vi "3. State Machine Based Traffic Light Simulator.vi"() -> ()   [LabVIEW 2018]
uses:
  Typedefs/States for State Machine based Example.ctl
panel:
  in  "stop":bool
  out "Yellow":bool
  out "Green":bool
  out "Red":bool
  out "Traffic Lights Picture":picture
  # "Traffic Light Graphic Vector by Vecteezy\n(https://www.vecteezy.com/free-vector/graphic)"
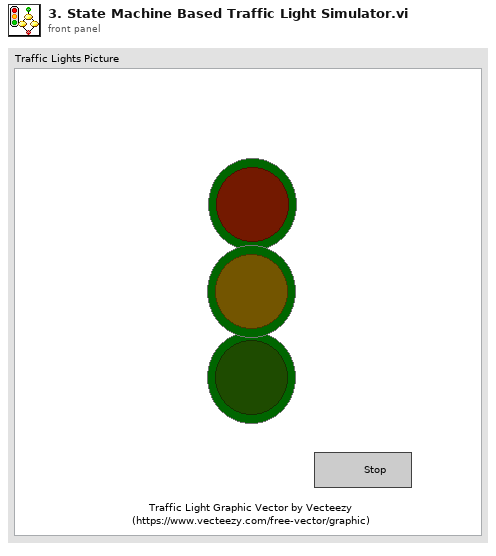
[diagram p1: front panel]
types:
  T1 = cluster{"Wait Before Red":u32, "Wait Before Yellow":u32, "Wait Before Green":u32}
  T2 = typedef "States for State Machine based Example.ctl" = enum16{"Initialize", "Red", "Yellow", "Green", "Wait Before Red", "Wait Before Yellow", "Wait Before Green", "Stop"}
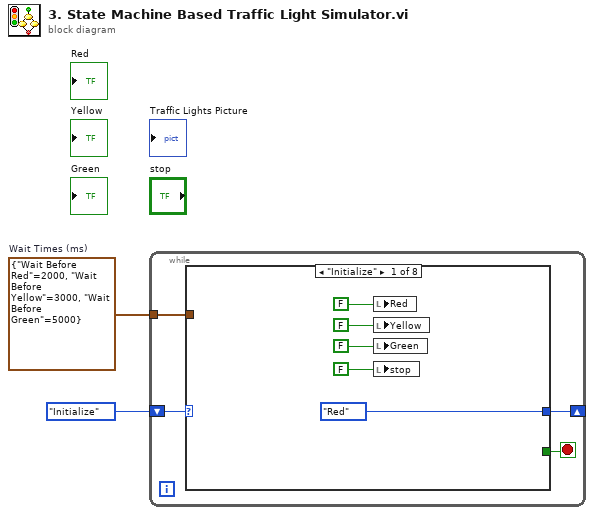
[diagram p0: block diagram]
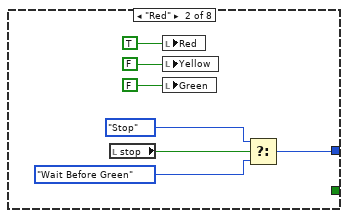
[diagram p2: hidden frame]
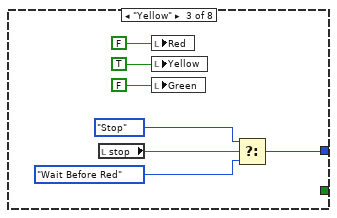
[diagram p3: hidden frame]
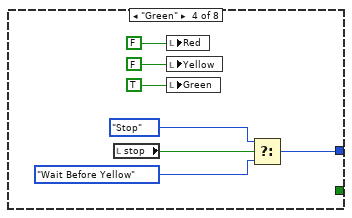
[diagram p4: hidden frame]
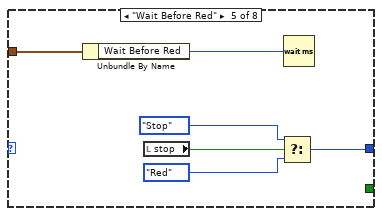
[diagram p5: hidden frame]
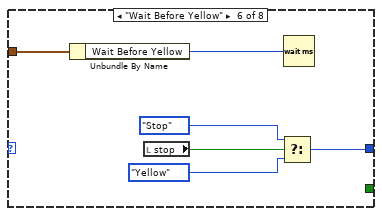
[diagram p6: hidden frame]
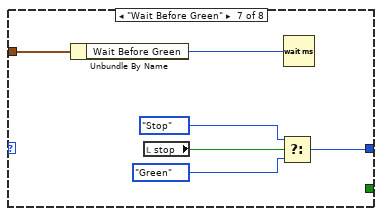
[diagram p7: hidden frame]
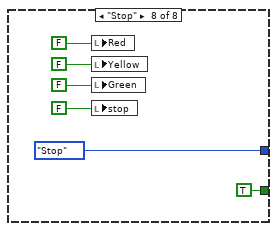
[diagram p8: hidden frame]
diagram:
  w1 = T1 {"Wait Before Red"=2000, "Wait Before Yellow"=3000, "Wait Before Green"=5000}  # Wait Times (ms)
  n1 = while {
    shift-right: [w5] -> _
    shift-left: States_for_State_Machine_based_Example."Initialize" -> [w6]
    tunnel: w1 -> [w4]
    stop <- w3 stop-if-true
    n2 = case shown="\"Initialize\"" w6 {
      tunnel: [States_for_State_Machine_based_Example."Red" w16 w23 w30 w37 w43 w49 States_for_State_Machine_based_Example."Stop"] -> w5
      tunnel: w4 -> [_ _ _ _ w34 w40 w46 _]
      tunnel: [_ _ _ _ _ _ _ TRUE] -> w3
      frame "Initialize" {
        n3 = local write "Red"(FALSE ("Red")) -> ()
        n4 = local write "Yellow"(FALSE ("Red")) -> ()
        n5 = local write "Green"(FALSE ("Red")) -> ()
        n6 = local write "stop"(FALSE ("stop")) -> ()
      }
      frame "Red" {
        n7 = local read "stop"() -> (w17:bool)
        n8 = local write "Red"(TRUE ("Red")) -> ()
        n9 = local write "Yellow"(FALSE ("Red")) -> ()
        n10 = local write "Green"(FALSE ("Red")) -> ()
        n11 = Select(t=States_for_State_Machine_based_Example."Stop", s=w17, f=States_for_State_Machine_based_Example."Wait Before Green") -> (s? t:f=w16:T2)
      }
      frame "Yellow" {
        n12 = local read "stop"() -> (w24:bool)
        n13 = local write "Red"(FALSE ("Red")) -> ()
        n14 = local write "Yellow"(TRUE ("Red")) -> ()
        n15 = local write "Green"(FALSE ("Red")) -> ()
        n16 = Select(t=States_for_State_Machine_based_Example."Stop", s=w24, f=States_for_State_Machine_based_Example."Wait Before Red") -> (s? t:f=w23:T2)
      }
      frame "Green" {
        n17 = local read "stop"() -> (w31:bool)
        n18 = local write "Red"(FALSE ("Red")) -> ()
        n19 = local write "Yellow"(FALSE ("Red")) -> ()
        n20 = local write "Green"(TRUE ("Red")) -> ()
        n21 = Select(t=States_for_State_Machine_based_Example."Stop", s=w31, f=States_for_State_Machine_based_Example."Wait Before Yellow") -> (s? t:f=w30:T2)
      }
      frame "Wait Before Red" {
        n22 = Unbundle By Name(w34) -> ("Wait Before Red"=w33:u32)
        n23 = local read "stop"() -> (w38:bool)
        n24 = Select(t=States_for_State_Machine_based_Example."Stop", s=w38, f=States_for_State_Machine_based_Example."Red") -> (s? t:f=w37:T2)
        n25 = Wait (ms)(milliseconds to wait=w33) -> ()  [unwired: 1 out]
      }
      frame "Wait Before Yellow" {
        n26 = Unbundle By Name(w40) -> ("Wait Before Yellow"=w39:u32)
        n27 = local read "stop"() -> (w44:bool)
        n28 = Select(t=States_for_State_Machine_based_Example."Stop", s=w44, f=States_for_State_Machine_based_Example."Yellow") -> (s? t:f=w43:T2)
        n29 = Wait (ms)(milliseconds to wait=w39) -> ()  [unwired: 1 out]
      }
      frame "Wait Before Green" {
        n30 = Unbundle By Name(w46) -> ("Wait Before Green"=w45:u32)
        n31 = local read "stop"() -> (w50:bool)
        n32 = Select(t=States_for_State_Machine_based_Example."Stop", s=w50, f=States_for_State_Machine_based_Example."Green") -> (s? t:f=w49:T2)
        n33 = Wait (ms)(milliseconds to wait=w45) -> ()  [unwired: 1 out]
      }
      frame "Stop" {
        n34 = local write "Red"(FALSE ("Red")) -> ()
        n35 = local write "Yellow"(FALSE ("Red")) -> ()
        n36 = local write "Green"(FALSE ("Red")) -> ()
        n37 = local write "stop"(FALSE ("stop")) -> ()
      }
    }
  }
